vi "Name.vi"(11 "Entity in":refnum<class "Entity.lvclass">) -> (2 "Name":string)   [LabVIEW 2020, in "Conditu2.lvlib" / "Entity.lvclass"]
uses:
  Entity.lvclass
  <vilib>/regexp/Match Regular Expression.xnode
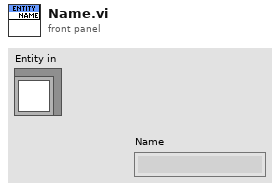
[diagram p1: front panel]
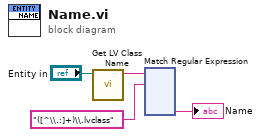
[diagram p0: block diagram]
diagram:
  n1 = call <vilib>:"Get LV Class Name.vi"("object"="Entity in") -> ("class name"=w3:string)  [unwired: 9 in, 1 out]
  n2 = xnode "Match Regular Expression"("input string"=w3, "regular expression"="([^\\.:]+)\\.lvclass") -> ("submatch 1"=→"Name":string)  [unwired: 4 in, 5 out]
